vi "Map URL.vi"(0 "Map Zoom":sgl=17.0, 1 "Current Latitude":dbl format="%#.6g", 2 "Current Longitude":dbl format="%#.6g", 3 "character":string="ATV", 5 "Y":dbl=570.0, 7 "X":dbl=350.0, 9 "Map Format":string(combo)="hybrid", 11 "Balloon String":string) -> (6 "URL":string)   [LabVIEW 2011]
panel:
  # "Start Position"
  # "Balloon Position"
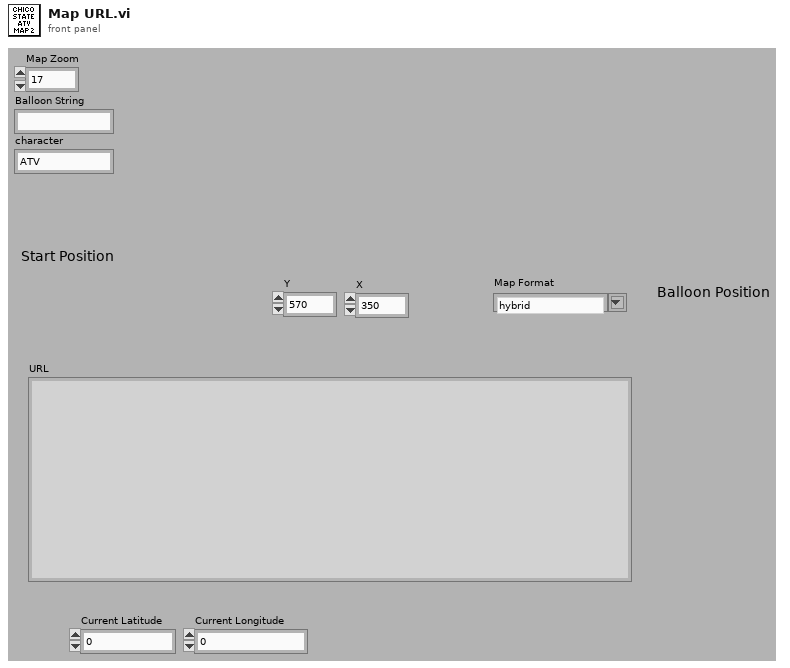
[diagram p1: front panel]
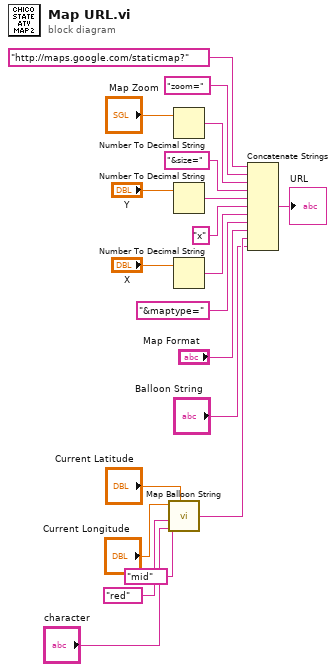
[diagram p0: block diagram]
diagram:
  n1 = call "Map Balloon String.vi"("Latitude"="Current Latitude", "character"="character", "color"="red", "size"="mid", "Longitude"="Current Longitude") -> ("Balloon"=w2:string)  [unwired: 1 in]
  n2 = Number To Decimal String(number="Map Zoom") -> (decimal integer string=w17:string)  [unwired: 1 in]
  n3 = Number To Decimal String(number="Y") -> (decimal integer string=w13:string)  [unwired: 1 in]
  n4 = Number To Decimal String(number="X") -> (decimal integer string=w11:string)  [unwired: 1 in]
  n5 = Concatenate Strings("http://maps.google.com/staticmap?" ("URL"), "zoom=", w17, "&size=", w13, "x", w11, "&maptype=", "Map Format", w2, "Balloon String") -> (→"URL":string)
